vi "FIRE CONTROL.vi"(8 "error in (no error)":errorcluster, 11 "control\ncluster":T1) -> (0 "error out":errorcluster, 3 "control\ncluster out":T1)   [LabVIEW 2023]
uses:
  ctrl defs/ctrl controllers.ctl
  Global stack names.vi
panel:
  in  "notes":string="Joystick 1- co-pilot\n\nINTAKE toggles intake rollers\n\nPUKE reverses intake & clears NOTE flag; timed to shut off\n\nFIRE starts firing sequence\n\nAMP toggles FLAP"
  in  "button for\nAMP":i32=3
  in  "button for\nFIRE":i32=2
  in  "button for\nPUKE":i32=1
  in  "button for\nINTAKE":i32=2
  out "Buttons":bool[](array[boolean])
  out "POVs":i16[](array[numeric])
  out "Axes":dbl[](array[numeric])
  in  "axis scale":dbl=0.7 format="%#_13g"
  in  "axis dead band":dbl=0.025 format="%#_13g"
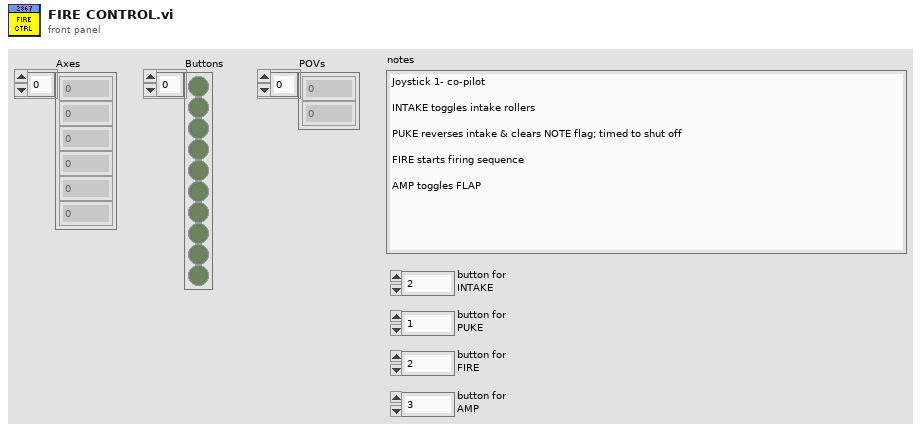
[diagram p1: front panel]
types:
  T1 = typedef "ctrl controllers.ctl" = cluster{"Axes":dbl[], "Buttons":bool[], "POVs":i16[]}
  T2 = typedef "ctrl stack - INTAKE SHOOTER.ctl" = cluster{"INTAKE STATE":string, "RUN INTAKE?":string, "RUN REVERSE?":string, "NOTE LOADED?":string, "SHOOTER STATE":string, "SHOOTER FIRE?":string, "SHOOT AMP?":string, "EXTEND FLAP?":string}
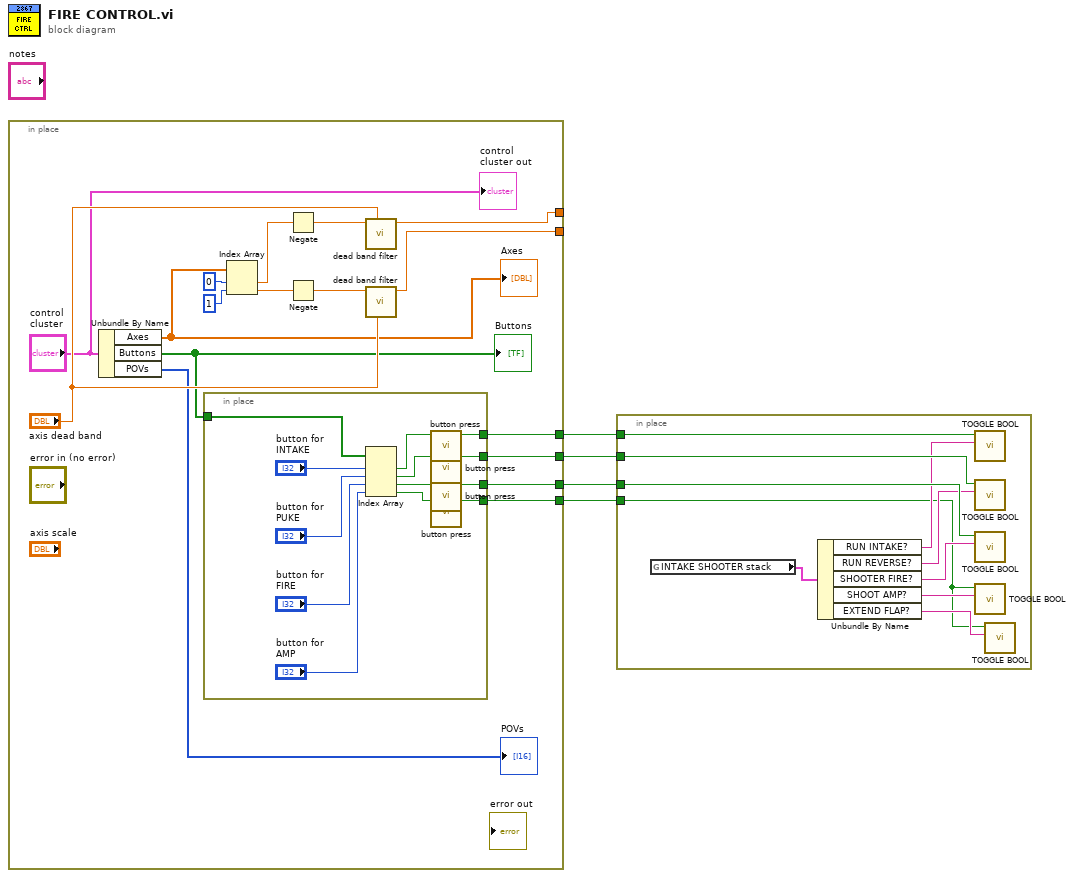
[diagram p0: block diagram]
diagram:
  n1 = in-place {
    in-place-border: [w14] -> _
    in-place-border: [w13] -> _
    in-place-border: [w8] -> w1
    in-place-border: [w7] -> w2
    in-place-border: [w6] -> w3
    in-place-border: [w5] -> w4
    n2 = Unbundle By Name("control\ncluster") -> ("Axes"=w11:dbl[], "Buttons"=w9:bool[], "POVs"=→"POVs":i16[])
    "Axes" <- w11
    "Buttons" <- w9
    n3 = in-place {
      in-place-border: w9 -> [w34]
      in-place-border: [w31] -> w8
      in-place-border: [w29] -> w7
      in-place-border: [w27] -> w6
      in-place-border: [w22] -> w5
      n4 = Index Array(array=w34, index #1="button for\nINTAKE", index #2="button for\nPUKE", index #3="button for\nFIRE", index #4="button for\nAMP") -> (element #1=w33:bool, element #2=w30:bool, element #3=w28:bool, element #4=w23:bool)
      n5 = call "button press.vi"("button IN"=w33) -> ("Button Pressed?"=w31:bool)  [unwired: 10 in]
      n6 = call "button press.vi"("button IN"=w30) -> ("Button Pressed?"=w29:bool)  [unwired: 10 in]
      n7 = call "button press.vi"("button IN"=w28) -> ("Button Pressed?"=w27:bool)  [unwired: 10 in]
      n8 = call "button press.vi"("button IN"=w23) -> ("Button Pressed?"=w22:bool)  [unwired: 10 in]
    }
    n9 = Index Array(array=w11, index #1=0 ("index"), index #2=1 ("index")) -> (element #1=w18:dbl, element #2=w17:dbl)
    n10 = Negate(x=w18) -> (-x=w16:dbl)
    n11 = Negate(x=w17) -> (-x=w15:dbl)
    n12 = call "dead band filter.vi"("deadband"="axis dead band", "input"=w16) -> ("output"=w14:dbl)  [unwired: 9 in]
    n13 = call "dead band filter.vi"("deadband"="axis dead band", "input"=w15) -> ("output"=w13:dbl)  [unwired: 9 in]
    "control\ncluster out" <- "control\ncluster"
  }
  n14 = in-place {
    in-place-border: w4 -> [w35]
    in-place-border: w3 -> [w41]
    in-place-border: w2 -> [w40]
    in-place-border: w1 -> [w38]
    n15 = global read "Global stack names.vi" "INTAKE SHOOTER stack"() -> (w44:T2)
    n16 = Unbundle By Name(w44) -> ("RUN INTAKE?"=w37:string, "RUN REVERSE?"=w39:string, "SHOOTER FIRE?"=w42:string, "SHOOT AMP?"=w43:string, "EXTEND FLAP?"=w36:string)
    n17 = call "TOGGLE BOOL.vi"("stack ref name"=w37, "Button Pressed?"=w38) -> ()  [unwired: 9 in, 1 out]
    n18 = call "TOGGLE BOOL.vi"("stack ref name"=w39, "Button Pressed?"=w40) -> ()  [unwired: 9 in, 1 out]
    n19 = call "TOGGLE BOOL.vi"("stack ref name"=w42, "Button Pressed?"=w41) -> ()  [unwired: 9 in, 1 out]
    n20 = call "TOGGLE BOOL.vi"("stack ref name"=w43, "Button Pressed?"=w35) -> ()  [unwired: 9 in, 1 out]
    n21 = call "TOGGLE BOOL.vi"("stack ref name"=w36, "Button Pressed?"=w35) -> ()  [unwired: 9 in, 1 out]
  }
